vi "GetMessages.vi"(0 "reference in":refnum<class "TelegramBOT.lvclass">, 5 "error in (no error)":errorcluster) -> (14 "reference out":refnum<class "TelegramBOT.lvclass">, 16 "Messages":T1[](array[typedef]), 17 "Connection":bool, 18 "ReceivedUpdates":i32, 19 "error out":errorcluster)   [LabVIEW 2014, in "TelegramBOT.lvclass"]
uses:
  TelegramBOT.lvclass
  MessageCluster.ctl
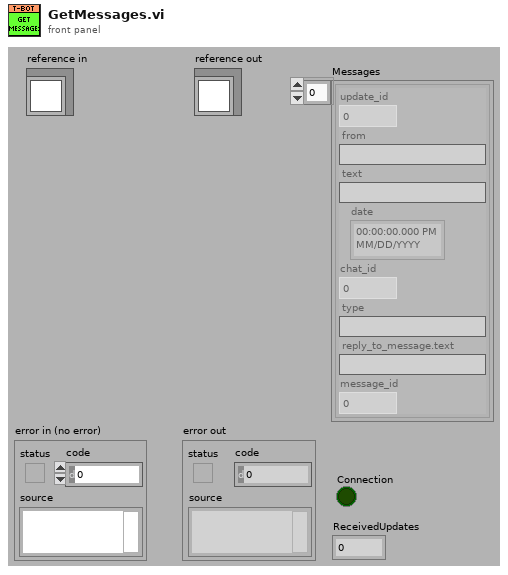
[diagram p1: front panel]
types:
  T1 = typedef "TelegramBOT.lvclass/MessageCluster.ctl" = cluster{"update_id":u32, "from":string, "text":string, "date":timestamp, "chat_id":i32, "type":string, "reply_to_message.text":string, "message_id":u32}
  T2 = typedef "TelegramBOT.lvclass/UpdateResultElem.ctl" = cluster{"update_id":u32, "message":cluster{"message_id":u32, "from":cluster{"id":u64, "first_name":string}, "chat":cluster{"id":i32, "first_name":string, "type":string}, "date":u32, "text":string, "reply_to_message":cluster{"message_id":u32, "from":cluster{"id":u64, "first_name":string}, "chat":cluster{"id":i32, "first_name":string, "type":string}, "date":u32, "text":string}}}
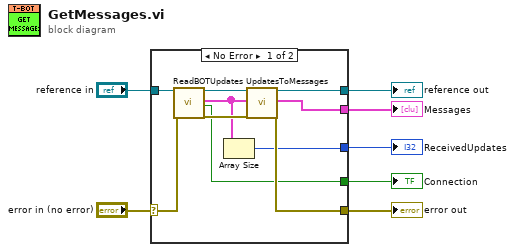
[diagram p0: block diagram]
diagram:
  n1 = case shown="No Error" "error in (no error)" {
    selector: "error in (no error)" -> [w16 w19]
    tunnel: [w12 w19] -> w6
    tunnel: [w14 w18] -> w4
    tunnel: "reference in" -> [w17 w18]
    tunnel: [w11 _] -> w3
    tunnel: [w10 _] -> w2
    tunnel: [w8 _] -> w1
    frame No Error {
      n2 = call "ReadBOTUpdates.vi"("reference in"=w17, "error in (no error)"=w16) -> ("reference out"=w15:refnum<class "TelegramBOT.lvclass">, "result"=w9:T2[], "Connection"=w11:bool, "error out"=w13:errorcluster)  [unwired: 14 in]
      n3 = Array Size(array=w9) -> (size(s)=w8:i32)
      n4 = call "UpdatesToMessages.vi"("reference in"=w15, "result"=w9, "error in (no error)"=w13) -> ("reference out"=w14:refnum<class "TelegramBOT.lvclass">, "Messages"=w10:T1[], "error out"=w12:errorcluster)  [unwired: 14 in]
    }
    frame Error {
    }
  }
  "error out" <- w6
  "reference out" <- w4
  "Connection" <- w3
  "Messages" <- w2
  "ReceivedUpdates" <- w1
